vi "CMD_SURVEY.vi"(6 "Gantry in":refnum<class "Gantry.lvclass">, 8 "error in (no error)":errorcluster, 10 "Arguments":string[](array[string]), 11 "gScript Interpreter in":refnum<class "gScript Interpreter.lvclass">) -> (0 "error out":errorcluster, 3 "gScript Interpreter out":refnum<class "gScript Interpreter.lvclass">, 4 "Gantry out":refnum<class "Gantry.lvclass">)   [LabVIEW 2024, in "gScript Interpreter.lvclass"]
uses:
  gScript Interpreter.lvclass
  Shared Components/Gantry Class/Gantry.lvclass
  gScript Interpreter.lvclass/gScript Interpreter.ctl
  Shared Components/FlexWorktable/FlexWorktable.lvclass
panel:
  out "Interuptor":bool
  in  "Interrupt Survey":bool
  out "Progress":u8(slide) scale=0.0..56.0
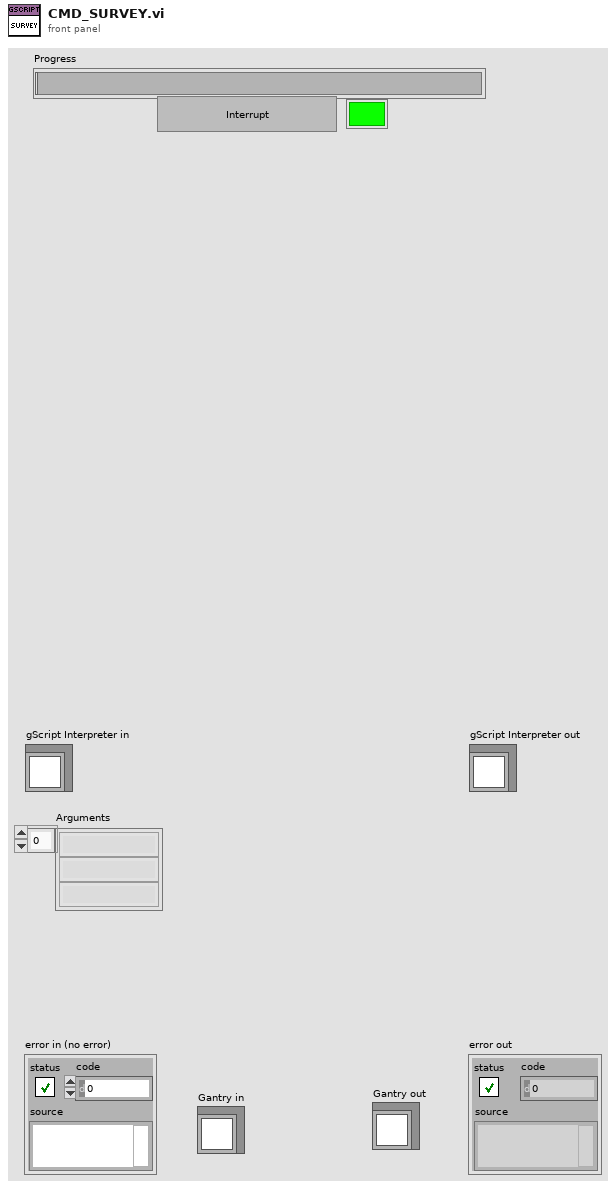
[diagram p1: front panel]
types:
  T1 = typedef "Memory Cell.ctl" = cluster{"type":T2, "x":dbl, "y":dbl, "z":dbl, "w":dbl}
  T2 = typedef "Memory Cell Type Enum.ctl" = enum16{"integer", "float", "vector", "rotation"}
  T3 = typedef "Physical Image.ctl" = cluster{"Image Position":refnum<class "Vec3d.lvclass">, "Image Reference":T4, "Field of View":cluster{"x(mm)":dbl, "y(mm)":dbl}}
  T4 = typedef "IMAQ Image.ctl" = refnum<image>
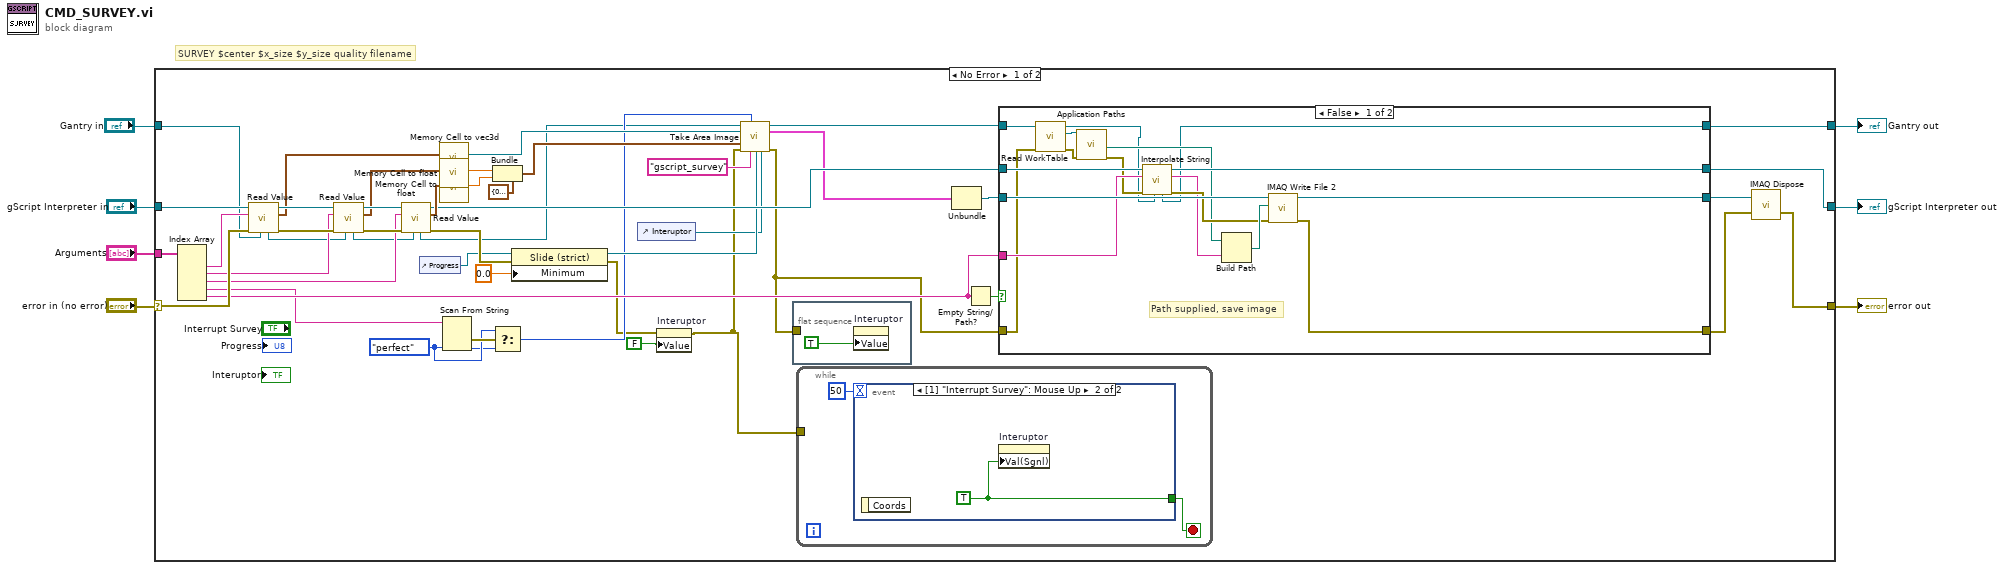
[diagram p0: block diagram]
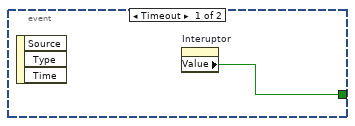
[diagram p2: hidden frame]
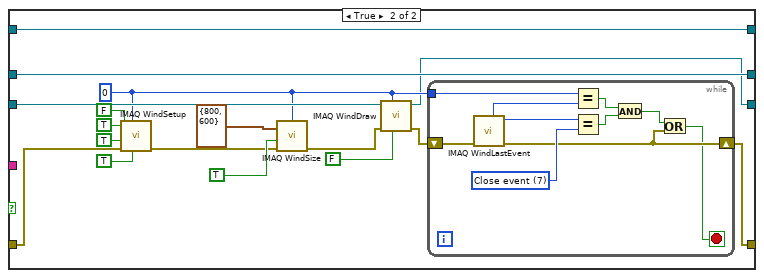
[diagram p3: hidden frame]
diagram:
  # "SURVEY $center $x_size $y_size quality filename"
  n1 = case shown="No Error" "error in (no error)" {
    selector: "error in (no error)" -> [w53 w107]
    tunnel: [w23 w107] -> w6
    tunnel: [w35 w106] -> w4
    tunnel: "gScript Interpreter in" -> [w54 w106]
    tunnel: "Arguments" -> [w55 _]
    tunnel: "Gantry in" -> [w16 w105]
    tunnel: [w39 w105] -> w1
    frame No Error {
      w19 = enum16{"perfect", "high", "medium", "low"}."perfect" ("Quality")
      n2 = Index Array(array=w55) -> (element #1=w42:string, element #2=w41:string, element #3=w40:string, element #4=w21:string, element #5=w22:string)  [unwired: 5 in]
      n3 = call-dynamic "Read Value.vi"("Gantry in"=w16, "error in (no error)"=w53, "String in"=w42, "gScript Interpreter in"=w54) -> ("error out"=w47:errorcluster, "Memory Cell"=w50:T1, "gScript Interpreter out"=w52:refnum<class "gScript Interpreter.lvclass">, "Gantry out"=w15:refnum<class "Gantry.lvclass">)  [unwired: 4 in]
      n4 = call-dynamic "Read Value.vi"("Gantry in"=w15, "error in (no error)"=w47, "String in"=w41, "gScript Interpreter in"=w52) -> ("error out"=w46:errorcluster, "Memory Cell"=w49:T1, "gScript Interpreter out"=w51:refnum<class "gScript Interpreter.lvclass">, "Gantry out"=w14:refnum<class "Gantry.lvclass">)  [unwired: 4 in]
      n5 = call-dynamic "Read Value.vi"("Gantry in"=w14, "error in (no error)"=w46, "String in"=w40, "gScript Interpreter in"=w51) -> ("error out"=w29:errorcluster, "Memory Cell"=w48:T1, "gScript Interpreter out"=w36:refnum<class "gScript Interpreter.lvclass">, "Gantry out"=w13:refnum<class "Gantry.lvclass">)  [unwired: 4 in]
      n6 = control-ref of="Progress"() -> (w27:refnum<vi>)
      n7 = call "Memory Cell to vec3d.vi"("Memory Cell"=w50) -> ("Vec3d out"=w28:refnum<class "Vec3d.lvclass">)  [unwired: 10 in]
      n8 = call "Memory Cell to float.vi"("Memory Cell"=w49) -> ("float out"=w44:dbl)  [unwired: 10 in]
      n9 = call "Memory Cell to float.vi"("Memory Cell"=w48) -> ("float out"=w43:dbl)  [unwired: 10 in]
      n10 = Scan From String(input string=w21, default 1=w19) -> (error out=w20:errorcluster, output 1=w18:enum16{"perfect", "high", "medium", "low"})  [unwired: 3 in, 2 out]
      n11 = Bundle(cluster=cluster{"Size-X(mm)":dbl, "Size-Y(mm)":dbl} {"Size-X(mm)"=0.0, "Size-Y(mm)"=0.0} ("Field of View"), "Size-X(mm)"=w44, "Size-Y(mm)"=w43) -> (w31:cluster{"Size-X(mm)":dbl, "Size-Y(mm)":dbl})
      n12 = Select(t=w19, s=w20, f=w18) -> (s? t:f=w17:enum16{"perfect", "high", "medium", "low"})
      n13 = property on="Property Node" class="Slide (strict)"(reference=w27, error in=w29, "Minimum"=0.0 ("Data Entry Limits:Minimum")) -> (reference out=w26:refnum<vi>, error out=w11:errorcluster)
      n14 = control-ref of="Interuptor"() -> (w9:refnum<vi>)
      n15 = property on="Interuptor" class="Bool (strict)"(error in=w11, "Value"=FALSE ("Interrupt Survey")) -> (error out=w8:errorcluster)  [unwired: 1 in, 1 out]
      n16 = call "Take Area Image.vi"("Gantry in"=w13, "Quality"=w17, "Image Center"=w28, "Field of View"=w31, "error in (no error)"=w8, "Image Name"="gscript_survey", "Slider Reference"=w26, "Interrupt Reference"=w9) -> ("Gantry out"=w34:refnum<class "Gantry.lvclass">, "Physical Image"=w33:T3, "error out"=w12:errorcluster)  [unwired: 5 in]
      n17 = flat-sequence {
        tunnel: w12 -> [_]
        frame #0 {
          n18 = property on="Interuptor" class="Bool (strict)"("Value"=TRUE ("Value (Signaling)")) -> ()  [unwired: 2 in, 2 out]
        }
      }
      n19 = while {
        tunnel: w8 -> [_]
        stop <- w58 stop-if-true
        n20 = event shown="[1] \"Interrupt Survey\": Mouse Up" {
          selector: _ -> [_ _]
          dyn-events: _ -> [_ _]
          timeout: 50 -> [_ _]
          tunnel: [w59 w60] -> w58
          event Timeout {
            n21 = event-data() -> ()  [unwired: 1 in, 3 out]
            n22 = property on="Interuptor" class="Bool (strict)"() -> ("Value"=w59:bool)  [unwired: 2 in, 2 out]
          }
          event "Interrupt Survey": Mouse Up {
            w60 = TRUE ("Interuptor")
            n23 = event-data() -> ()  [unwired: 1 in, 1 out]
            n24 = property on="Interuptor" class="Bool (strict)"("Val(Sgnl)"=w60) -> ()  [unwired: 2 in, 2 out]
          }
        }
      }
      n25 = Unbundle(w33) -> ("Image Reference"=w37:T4)  [unwired: 2 out]
      n26 = Empty String/Path?(string/path=w22) -> (empty?=w38:bool)
      n27 = case shown="False" w38 {
        tunnel: w34 -> [w68 w94]
        tunnel: w12 -> [w67 w88]
        tunnel: w37 -> [w77 w92]
        tunnel: w22 -> [w70 _]
        tunnel: [w62 w94] -> w39
        tunnel: [w75 w79] -> w25
        tunnel: [w74 w78] -> w24
        tunnel: w36 -> [w73 w93]
        tunnel: [w71 w93] -> w35
        frame False {
          # "Path supplied, save image"
          n28 = call-dynamic "Read WorkTable.vi"("error in"=w67, "Gantry Class in"=w68) -> ("error out"=w61:errorcluster, "Worktable"=w66:refnum<class "FlexWorktable.lvclass">, "Gantry Class out"=w63:refnum<class "Gantry.lvclass">)  [unwired: 7 in]
          n29 = call "Application Paths.vi"("FlexWorktable in"=w66, "error in (no error)"=w61) -> ("Logs Path"=w65:path, "error out"=w64:errorcluster)  [unwired: 11 in, 5 out]
          n30 = call-dynamic "Interpolate String.vi"("Gantry in"=w63, "error in (no error)"=w64, "Input String"=w70, "gScript Interpreter in"=w73) -> ("error out"=w72:errorcluster, "Output String"=w69:string, "gScript Interpreter out"=w71:refnum<class "gScript Interpreter.lvclass">, "Gantry out"=w62:refnum<class "Gantry.lvclass">)  [unwired: 4 in]
          n31 = Build Path(base path=w65, name or relative path=w69) -> (appended path=w76:path)
          n32 = call-poly "IMAQ Write File 2"("error in (no error)"=w72, "File Path"=w76, "Image"=w77) -> ("error out"=w74:errorcluster, "Image Out (duplicate)"=w75:T4)  [unwired: 7 in]
        }
        frame True {
          w80 = 0 ("Window Number (0...15)")
          n33 = call "IMAQ WindSetup"("Window is floating? (No)"=TRUE, "Window Number (0...15)"=w80, "error in (no error)"=w88, "Window has title bar? (Yes)"=TRUE, "Window can close? (Yes)"=TRUE, "Window can grow? (Yes)"=FALSE) -> ("error out"=w87:errorcluster)  [unwired: 5 in]
          n34 = call "IMAQ WindSize"("error in (no error)"=w87, "Scrollbars? (N)"=TRUE, "Width & Height"=cluster{"Width":i32, "Height":i32} {"Width"=800, "Height"=600}, "Window Number"=w80) -> ("error out"=w91:errorcluster)  [unwired: 2 in, 2 out]
          n35 = call "IMAQ WindDraw"("Resize to Image Size? (Y)"=FALSE, "Window Number (0...15)"=w80, "error in (no error)"=w91, "Image"=w92) -> ("error out"=w81:errorcluster, "Image Out (duplicate)"=w79:T4)  [unwired: 6 in]
          n36 = while {
            shift-right: [w96] -> w78
            shift-left: w81 -> [w104]
            tunnel: w80 -> [w103]
            stop <- w95 stop-if-true
            w100 = 7 items=["No  event", "Click event", "Draw event", "Move event", "Size event", "Scroll event", "Activate event", "Close event", "Double click event"] ("Event")
            n37 = call "IMAQ WindLastEvent"("error in (no error)"=w104) -> ("error out"=w96:errorcluster, "Event"=w101:i32, "Window Number (0...15)"=w102:i32)  [unwired: 5 in, 3 out]
            n38 = Equal?(x=w103, y=w102) -> (x = y?=w99:bool)
            n39 = Equal?(x=w101, y=w100) -> (x = y?=w98:bool)
            n40 = And(x=w99, y=w98) -> (x .and. y?=w97:bool)
            n41 = Or(x=w97, y=w96) -> (x .or. y?=w95:bool)
          }
        }
      }
      n42 = call "IMAQ Dispose"("Image"=w25, "error in (no error)"=w24) -> ("error out"=w23:errorcluster)  [unwired: 4 in]
    }
    frame Error {
    }
  }
  "error out" <- w6
  "gScript Interpreter out" <- w4
  "Gantry out" <- w1
